vi "Global.vi"() -> ()   [LabVIEW 2015]
panel:
  out "Ion Sniffer Version":string
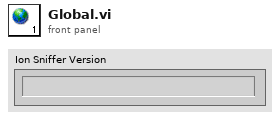
[diagram p1: front panel]
diagram:
